vi "InspectCallCleanup.vi"(6 "Error":errorcluster, 7 "Actor":refnum<class "Actor.lvclass">, 10 "PreInspectCallError":errorcluster, 11 "Message":refnum<class "Msg.lvclass">) -> (3 "Message":refnum<class "Msg.lvclass">, 4 "Error":errorcluster, 5 "Actor":refnum<class "Actor.lvclass">)   [LabVIEW 2020, in "_Template.lvlib" / "{{Actor}}.lvlib" / "Actor.lvclass"]
uses:
  jettl/jettl/Msg/Msg.lvclass
  Actor.lvclass
  Actor.lvclass/Actor.ctl
  jettl/jettl/Actor/Actor.lvclass
panel:
  # "This front panel should not be manipulated."
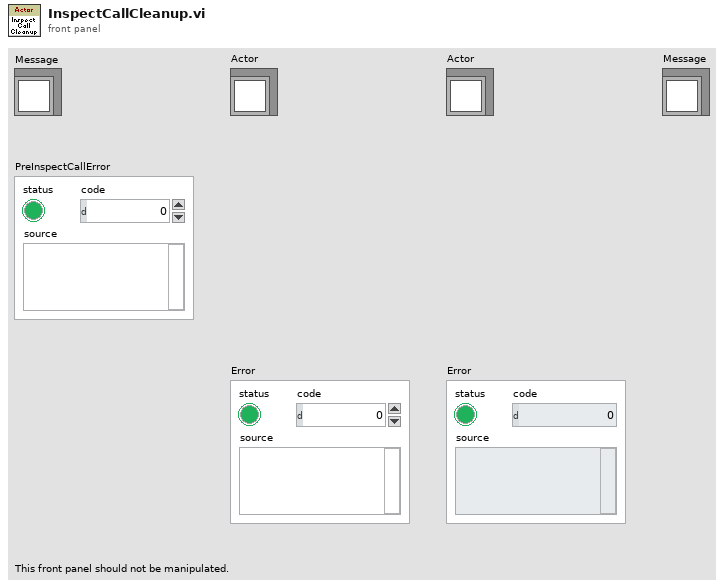
[diagram p1: front panel]
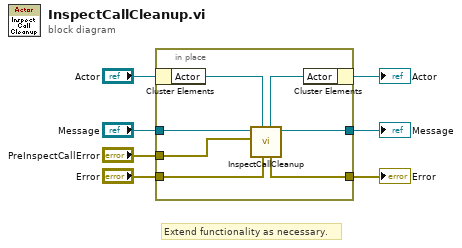
[diagram p0: block diagram]
diagram:
  # "Extend functionality as necessary."
  n1 = in-place {
    in-place-border: "Message" -> [w12]
    in-place-border: [w11] -> w4
    in-place-border: [w10] -> w3
    in-place-border: "Error" -> [w9]
    in-place-border: "PreInspectCallError" -> [w8]
    n2 = in-place-cluster #1("Actor") -> ("Actor"=w14:refnum<class "Actor.lvclass">)
    n3 = call-dynamic "InspectCallCleanup.vi"("Error"=w9, "Actor"=w14, "PreInspectCallError"=w8, "Message"=w12) -> ("Message"=w11:refnum<class "Msg.lvclass">, "Error"=w10:errorcluster, "Actor"=w13:refnum<class "Actor.lvclass">)  [unwired: 5 in]
    n4 = in-place-cluster #1("Actor"=w13) -> (→"Actor":refnum<class "Actor.lvclass">)
  }
  "Error" <- w3
  "Message" <- w4
